vi "data_visualize.vi"() -> ()   [LabVIEW 2013]
panel:
  out "Final Trap Depth (uK)":string
  out "Final Trap Depth (V)":string
  out "ODT Evaporation Trajectory":dbl[](graph)
  in  "?":bool
  out "Atom Cloud Fits":dbl[][](graph)
  out "Pico Scope Channel B":T1(graph)
  out "Pico Scope Channel A":T1(graph)
  out "MCS Sum":u32[](graph)
  out "MCS Counts Out":u32[][](graph)
  out "Temperature (K) y":dbl=7.671884209450556e-07 format="%#_6p"
  out "Temperature (K) x":dbl=7.730172326594958e-07 format="%#_6p"
  out "Number":dbl=355885.42342174763 format="%^#_6g"
  out "Temperature Vs Time":dbl(graph)=355885.42342174763 caption="Waveform Chart"
  out "Number Vs Time":dbl(graph)=355885.42342174763 caption="Waveform Chart"
  out "ROI OD":dbl[][](graph)
  out "Atoms - BG":dbl[][](graph)
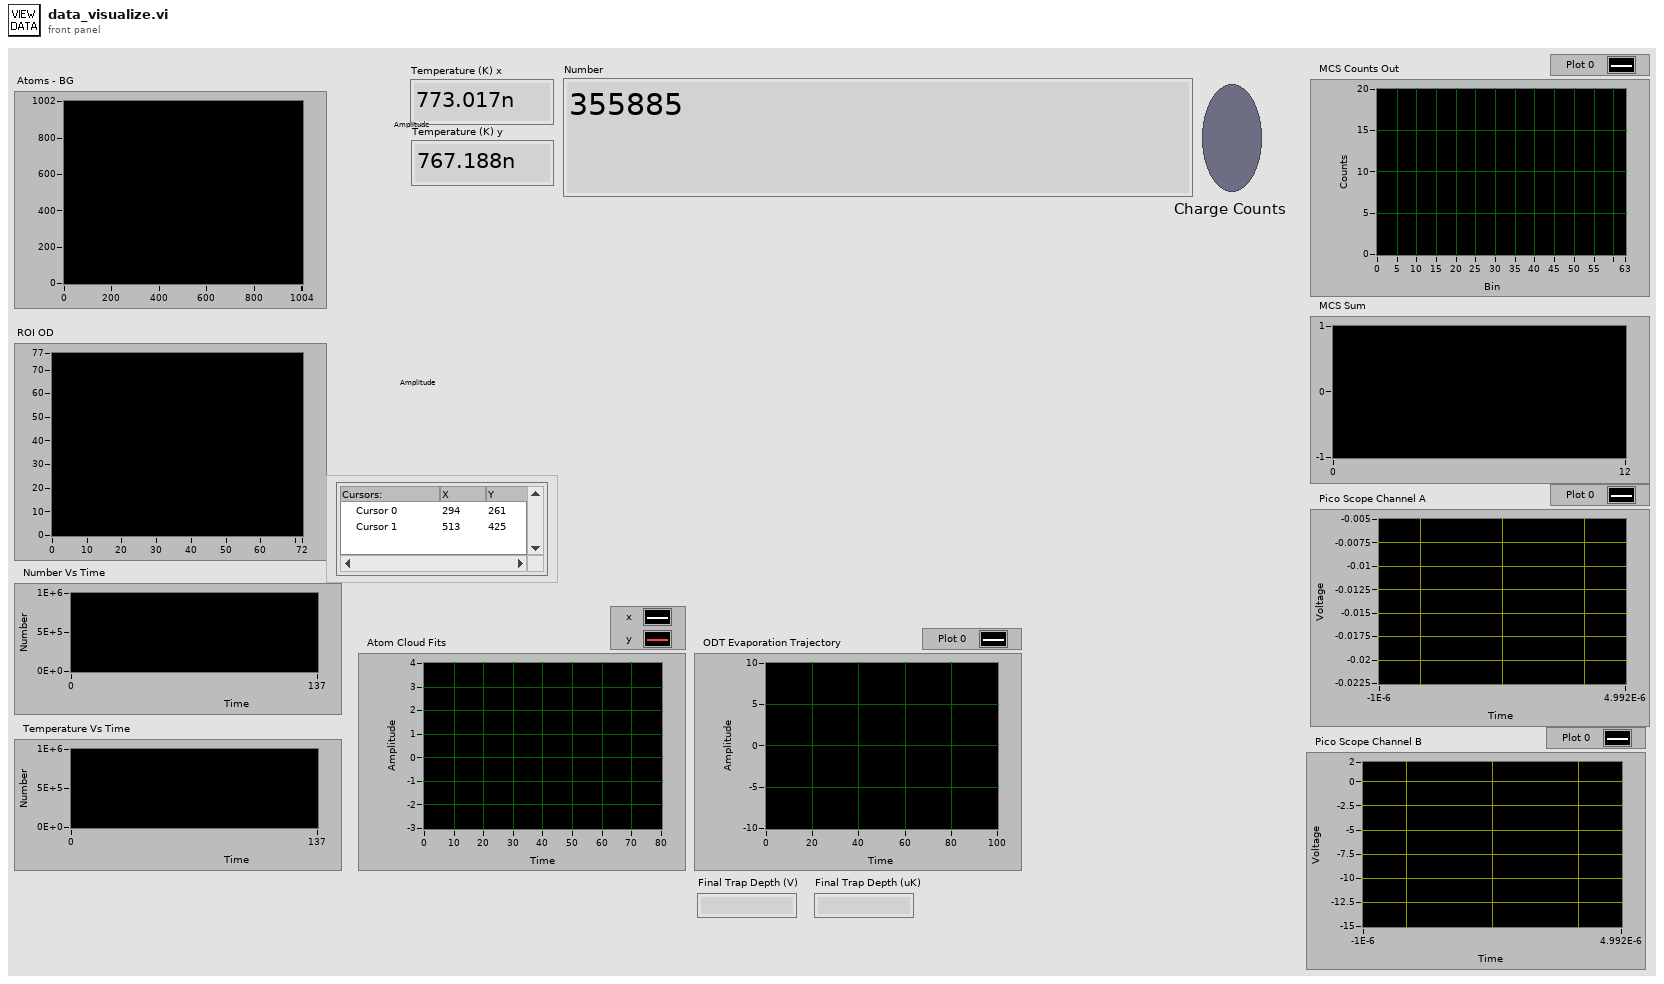
[diagram p1: front panel]
types:
  T1 = cluster{"Channel A Out":dbl[], "Channel A Out":dbl[]}[]
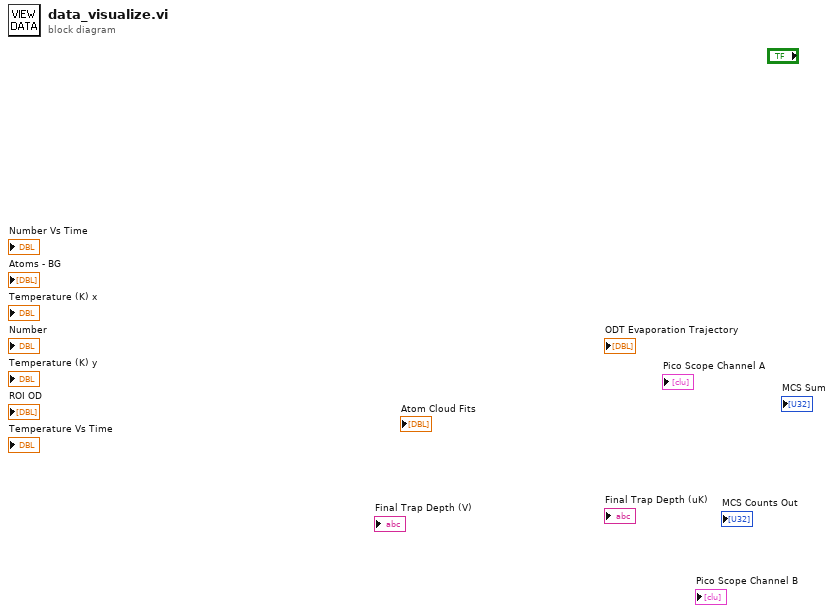
[diagram p0: block diagram]
diagram:
